vi "CreateMultiPointMultiChannelArray.vi"(8 "error in (no error)":errorcluster, 11 "MultiChannelSamplesIn":dbl[][](array[numeric]) format="%0.2f") -> (0 "error out":errorcluster, 3 "MultiPointReadingArrayOut":T1)   [LabVIEW 2014, in "SamplerPlugins.lvlib" / "NiPxi6123.lvclass"]
uses:
  NiPxi6123.lvclass
  NISTSamplerPluginsBaseClass/TypeDefs/MultiPointReadingArrayParams.ctl
  NISTSamplerPluginsBaseClass/TypeDefs/MultiPointReadingParams.ctl
  NISTSamplerPluginsBaseClass/SamplerPluginsBase.lvclass
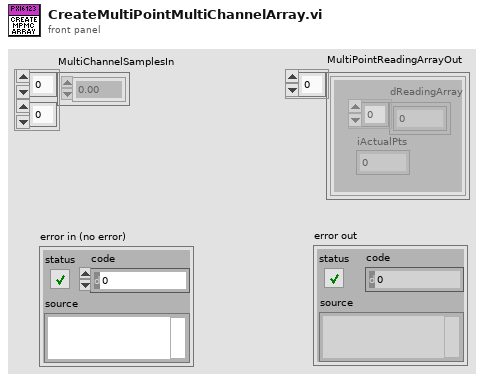
[diagram p1: front panel]
types:
  T1 = typedef "SamplerPlugins.lvlib/SamplerPluginsBase.lvclass/MultiPointReadingArrayParams.ctl" = cluster{"dReadingArray":dbl[], "iActualPts":i32}[]
  T2 = typedef "SamplerPlugins.lvlib/SamplerPluginsBase.lvclass/MultiPointReadingParams.ctl" = cluster{"dReadingArray":dbl[], "iActualPts":i32}
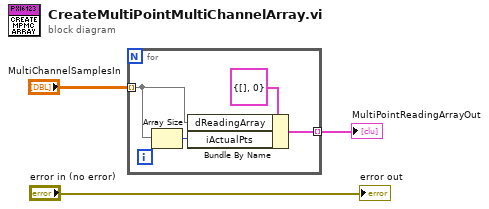
[diagram p0: block diagram]
diagram:
  n1 = for {
    tunnel: "MultiChannelSamplesIn" -> [w5] mode=indexing
    tunnel: [w4] -> w2 mode=indexing
    n2 = Array Size(array=w5) -> (size(s)=w6:i32)
    n3 = Bundle By Name(cluster=T2 {"dReadingArray"=[], "iActualPts"=0} ("MultiPointReadingParams"), "dReadingArray"=w5, "iActualPts"=w6) -> (w4:T2)
  }
  "MultiPointReadingArrayOut" <- w2
  "error out" <- "error in (no error)"
